vi "BoP Input Client.vi"() -> ()   [LabVIEW 2017]
uses:
  <vilib>/OPCUA/controls/Write Status.ctl
  <vilib>/OPCUA/controls/NodeId.ctl
  <vilib>/OPCUA/client/Multiple Write Double Array.vi
  <vilib>/OPCUA/NI OPC UA Client.lvlib
panel:
  in  "Stop BoP Input Writing":bool
  in  "Time Stamp":timestamp
  in  "Node Status":T1 items=["Good"=0, "Uncertain_InitialValue"=1083310080, "Uncertain_LastUsableValue"=1083179008, "Uncertain_SensorNotAccurate"=1083375616, "Uncertain_EngineeringUnitsExceeded"=1083441152, "Bad_NoCommunication"=2150694912, "Bad_NotReadable"=2151284736, "Bad_NotWritable"=2151350272, "Bad_OutOfRange"=2151415808, "Bad_WaitingForInitialData"=2150760448]
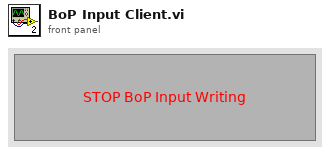
[diagram p1: front panel]
types:
  T1 = typedef "Write Status.ctl" = u32
  T2 = cluster{"message mode":enum16{"None", "Sign", "Sign and Encrypt"}, "security":enum16{"Basic256", "Basic128Rsa15"}}
  T3 = typedef "OPC UA Client Refnum.ctl" = refnum<k21>
  T4 = typedef "NodeId.ctl" = string
  T5 = cluster{"node ID":T4, "value":dbl[], "timestamp (current time)":timestamp, "node status":T1}
  T6 = cluster{"node ID":T4, "value":dbl[], "timestamp (current time)":timestamp, "node status":T1}[]
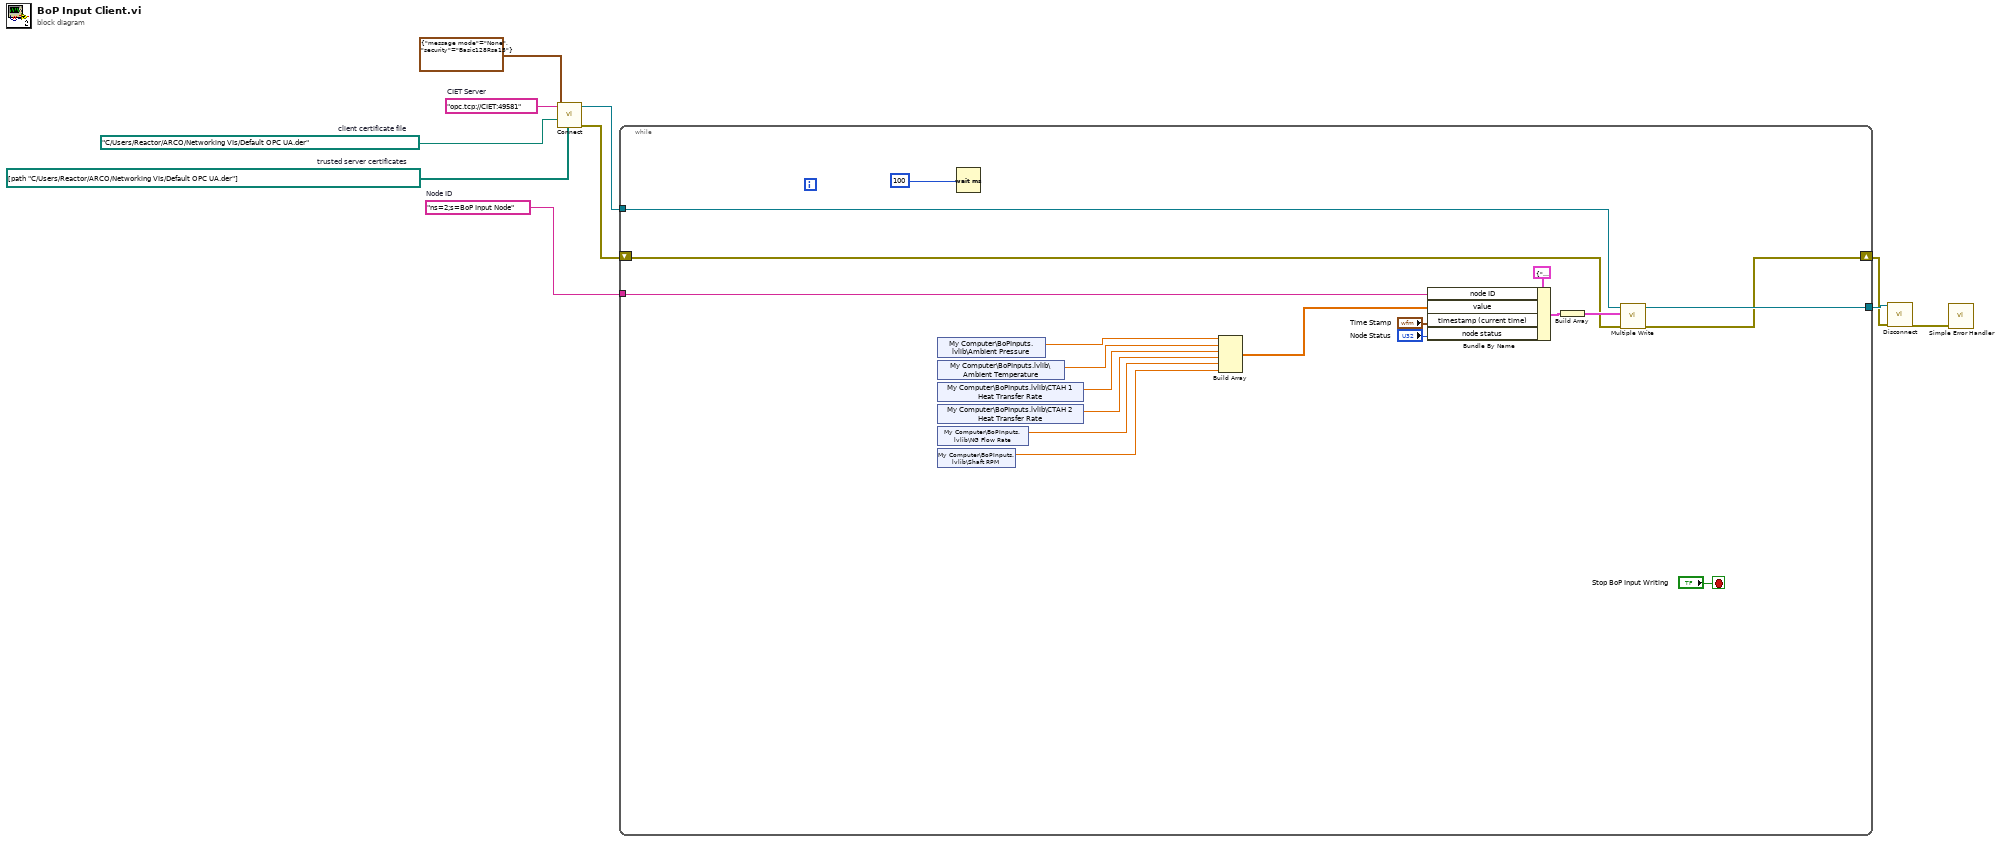
[diagram p0: block diagram]
diagram:
  w4 = path[] [path "C:/Users/Reactor/ARCO/Networking VIs/Default OPC UA.der"]  # trusted server certificates
  w5 = path "C:/Users/Reactor/ARCO/Networking VIs/Default OPC UA.der"  # client certificate file
  w7 = "ns=2;s=BoP Input Node"  # Node ID
  w9 = "opc.tcp://CIET:49581"  # CIET Server
  n1 = call <vilib>:"Connect.vi"("trusted server certificates"=w4, "client certificate file"=w5, "security policy"=T2 {"message mode"=enum."None", "security"=enum."Basic128Rsa15"}, "server endpoint URL"=w9) -> ("error out"=w2:errorcluster, "OPC UA client refnum out"=w8:T3)  [unwired: 5 in, 1 out]
  n2 = while {
    tunnel: w7 -> [w28]
    tunnel: w8 -> [w26]
    tunnel: [w27] -> w6
    shift-right: [w20] -> w1
    shift-left: w2 -> [w19]
    stop <- "Stop BoP Input Writing" stop-if-true
    n3 = shared-variable "My Computer\\BoPInputs.lvlib\\Ambient Pressure"() -> (w17:sgl)  [unwired: 1 in, 1 out]
    n4 = shared-variable "My Computer\\BoPInputs.lvlib\\Ambient Temperature"() -> (w16:sgl)  [unwired: 1 in, 1 out]
    n5 = shared-variable "My Computer\\BoPInputs.lvlib\\CTAH 1 Heat Transfer Rate"() -> (w15:sgl)  [unwired: 1 in, 1 out]
    n6 = shared-variable "My Computer\\BoPInputs.lvlib\\CTAH 2 Heat Transfer Rate"() -> (w14:sgl)  [unwired: 1 in, 1 out]
    n7 = shared-variable "My Computer\\BoPInputs.lvlib\\NG Flow Rate"() -> (w13:sgl)  [unwired: 1 in, 1 out]
    n8 = shared-variable "My Computer\\BoPInputs.lvlib\\Shaft RPM"() -> (w12:sgl)  [unwired: 1 in, 1 out]
    n9 = Wait (ms)(milliseconds to wait=u32 100) -> ()  [unwired: 1 out]
    n10 = Build Array(w17, w16, w15, w14, w13, w12) -> (w11:sgl[])
    n11 = Bundle By Name(cluster=T5 {"node ID"="", "value"=[], "timestamp (current time)"=timestamp(0 s since 1904-01-01), "node status"=0} ("request"), "node ID"=w28, "value"=w11, "timestamp (current time)"="Time Stamp", "node status"="Node Status") -> (w22:T5)
    n12 = Build Array(w22) -> (w21:T6)
    n13 = call-poly <vilib>:"Multiple Write.vi"("error in (no error)"=w19, "requests"=w21, "OPC UA client refnum in"=w26) -> ("error out"=w20:errorcluster, "OPC UA client refnum out"=w27:T3)  [unwired: 5 in, 2 out]
  }
  n14 = call <vilib>:"Disconnect.vi"("error in (no error)"=w1, "OPC UA client refnum in"=w6) -> ("error out"=w10:errorcluster)  [unwired: 9 in]
  n15 = call <vilib>:"Simple Error Handler.vi"("error in (no error)"=w10) -> ()  [unwired: 4 in, 5 out]
